vi "RNN.vi"(3 "Input 2":u16, 4 "Input 1":u16, 5 "Weights":sgl[](array[numeric])) -> (0 "Downwards":u16, 1 "Still":u16, 2 "Upwards":u16)   [LabVIEW 2020]
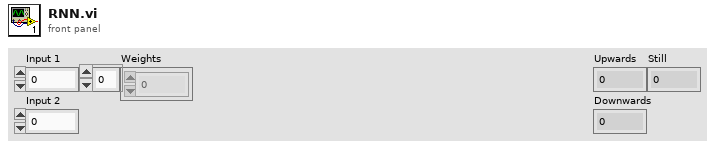
[diagram p1: front panel]
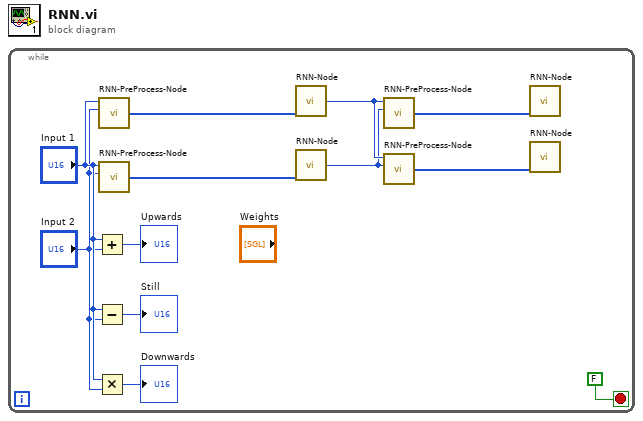
[diagram p0: block diagram]
diagram:
  n1 = while {
    stop <- FALSE stop-if-true
    n2 = Add(x="Input 1", y="Input 2") -> (x+y=→"Upwards":u16)
    n3 = Subtract(x="Input 1", y="Input 2") -> (x-y=→"Still":u16)
    n4 = Multiply(x="Input 1", y="Input 2") -> (x*y=→"Downwards":u16)
    n5 = call "RNN-PreProcess-Node.vi"("Input 2"="Input 2", "Input"="Input 1") -> ("Output"=w11:i16[])  [unwired: 4 in]
    n6 = call "RNN-PreProcess-Node.vi"("Input 2"="Input 2", "Input"="Input 1") -> ("Output"=w6:i16[])  [unwired: 4 in]
    n7 = call "RNN-Node.vi"("Input_Array"=w11) -> ("Output"=w2:i16)  [unwired: 4 in]
    n8 = call "RNN-Node.vi"("Input_Array"=w6) -> ("Output"=w1:i16)  [unwired: 4 in]
    n9 = call "RNN-PreProcess-Node.vi"("Input 2"=w1, "Input"=w2) -> ("Output"=w7:i16[])  [unwired: 4 in]
    n10 = call "RNN-PreProcess-Node.vi"("Input 2"=w1, "Input"=w2) -> ("Output"=w5:i16[])  [unwired: 4 in]
    n11 = call "RNN-Node.vi"("Input_Array"=w7) -> ()  [unwired: 4 in, 1 out]
    n12 = call "RNN-Node.vi"("Input_Array"=w5) -> ()  [unwired: 4 in, 1 out]
  }
